vi "Act System RT main.vi"() -> ()   [LabVIEW 2014]
uses:
  <vilib>/myRIO/Instrument Drivers/Onboard IO/PWM/typedefs/PWM Reference.ctl
  <vilib>/myRIO/Common/Instrument Driver Framework/Utilities/typedefs/myRIO Generic Hardware Reference.ctl
  <vilib>/myRIO/Common/Instrument Driver Framework/Utilities/typedefs/Hardware Version Enum.ctl
  <vilib>/myRIO/Common/Instrument Driver Framework/Utilities/typedefs/myRIO v1.0 Reference.ctl
  <vilib>/myRIO/Common/Instrument Driver Framework/Utilities/typedefs/Generic FPGA Reference.ctl
  <vilib>/myRIO/Common/Instrument Driver Framework/myRIO v1.0/PWM/typedefs/PWM Channels Enum.ctl
  <vilib>/myRIO/Instrument Drivers/Onboard IO/PWM/typedefs/PWM Configuration.ctl
  <vilib>/userdefined/High Color/nirio_resource_hc.ctl
  <vilib>/myRIO/Instrument Drivers/Onboard IO/AI/typedefs/AI Reference.ctl
  <vilib>/myRIO/Common/Instrument Driver Framework/myRIO v1.0/AI/typedefs/AI Channels List.ctl
  <vilib>/myRIO/Common/Instrument Driver Framework/myRIO v1.0/AI/typedefs/AI Channels Enum.ctl
  <vilib>/myRIO/Common/Instrument Driver Framework/Utilities/typedefs/Analog Scaling Constants List.ctl
  <vilib>/myRIO/Common/Instrument Driver Framework/Utilities/typedefs/Analog Scaling Constants.ctl
  <vilib>/myRIO/Common/Instrument Driver Framework/myRIO v1.0/PWM/vis/myRIO v1.1 Open PWM.vi
  <vilib>/myRIO/Common/Instrument Driver Framework/myRIO v1.0/AI/vis/myRIO v1.1 Open AI.vi
  <vilib>/myRIO/Common/Instrument Driver Framework/Utilities/vis/Validate Channels.vi
  <vilib>/myRIO/Common/Instrument Driver Framework/myRIO v1.0/PWM/vis/myRIO v1.0 Reserve PWM.vi
  <vilib>/myRIO/Instrument Drivers/Onboard IO/PWM/vis/Set Duty Cycle and Frequency.vi
  <vilib>/myRIO/Common/Instrument Driver Framework/myRIO v1.0/AI/vis/myRIO v1.0 Reserve AI.vi
  <vilib>/myRIO/Common/Instrument Driver Framework/myRIO v1.0/DIO/vis/myRIO v1.1 Open DIO.vi
  <vilib>/myRIO/Common/Instrument Driver Framework/myRIO v1.0/PWM/vis/myRIO v1.0 Close PWM.vi
  <vilib>/myRIO/Common/Instrument Driver Framework/myRIO v1.0/AI/vis/myRIO v1.0 Close AI.vi
  <vilib>/myRIO/Common/Instrument Driver Framework/myRIO v1.0/DIO/vis/myRIO v1.0 Close DIO.vi
  <vilib>/myRIO/Common/Instrument Driver Framework/myRIO v1.0/PWM/vis/myRIO v1.0 Build MUX Configuration PWM.vi
  <vilib>/myRIO/Common/Instrument Driver Framework/myRIO v1.0/Resource Manager/vis/myRIO v1.0 Reserve Channel List.vi
  <vilib>/myRIO/Common/Instrument Driver Framework/myRIO v1.0/AI/vis/myRIO v1.0 Build MUX Configuration AI.vi
  <vilib>/myRIO/Common/Instrument Driver Framework/myRIO v1.0/DIO/vis/myRIO v1.0 Reserve DIO.vi
  <vilib>/myRIO/Common/Instrument Driver Framework/myRIO v1.0/PWM/vis/myRIO v1.0 Unreserve PWM.vi
  <vilib>/myRIO/Common/Instrument Driver Framework/myRIO v1.0/AI/vis/myRIO v1.0 Unreserve AI.vi
  <vilib>/myRIO/Common/Instrument Driver Framework/myRIO v1.0/DIO/vis/myRIO v1.0 Unreserve DIO.vi
  <vilib>/myRIO/Common/Instrument Driver Framework/myRIO v1.0/Resource Manager/vis/myRIO v1.0 Create Configuration List.vi
  <vilib>/myRIO/Common/Instrument Driver Framework/myRIO v1.0/Resource Manager/vis/myRIO v1.0 Reserve Channel.vi
  <vilib>/myRIO/Common/Instrument Driver Framework/myRIO v1.0/Resource Manager/vis/myRIO v1.0 Unreserve Channel.vi
  <vilib>/myRIO/Common/Instrument Driver Framework/myRIO v1.0/DIO/vis/myRIO v1.0 Build MUX Configuration DIO.vi
  <vilib>/myRIO/Common/Instrument Driver Framework/myRIO v1.0/Resource Manager/vis/myRIO v1.0 Unreserve Channel List.vi
  <vilib>/myRIO/Common/Instrument Driver Framework/myRIO v1.0/Resource Manager/vis/myRIO v1.0 Build Mutex Name.vi
  <vilib>/Utility/VariantDataType/GetNumericInfo.vi
  <vilib>/Utility/error.llb/Error Cluster From Error Code.vi
  <vilib>/myRIO/Common/Instrument Driver Framework/myRIO v1.0/myRIO v1.1 Open.vi
  <vilib>/myRIO/Common/Instrument Driver Framework/Utilities/vis/IO Manager.vi
  <vilib>/myRIO/Common/Instrument Driver Framework/Utilities/vis/Configuration Manager.vi
  <vilib>/myRIO/Common/Instrument Driver Framework/myRIO v1.0/Resource Manager/vis/myRIO v1.0 Configure IO.vi
  <vilib>/myRIO/Common/Instrument Driver Framework/myRIO v1.0/myRIO v1.0 Close.vi
  <vilib>/myRIO/Common/Instrument Driver Framework/myRIO v1.0/AI/vis/myRIO v1.0 Get Scaling Constants AI.vi
  <vilib>/myRIO/Common/Instrument Driver Framework/myRIO v1.0/PWM/vis/myRIO v1.0 Write PWM.vi
  <vilib>/myRIO/Common/Instrument Driver Framework/myRIO v1.0/PWM/vis/myRIO v1.0 Shutdown PWM.vi
  <vilib>/myRIO/Common/Instrument Driver Framework/myRIO v1.0/AI/vis/myRIO v1.0 Read AI.vi
  <vilib>/myRIO/Common/Instrument Driver Framework/myRIO v1.0/DIO/vis/myRIO v1.0 Write DIO.vi
  <vilib>/myRIO/Common/Instrument Driver Framework/myRIO v1.0/DIO/vis/myRIO v1.0 Shutdown DIO.vi
  <vilib>/myRIO/Instrument Drivers/Onboard IO/AI/vis/myRIO AI Open.xnode
  <vilib>/myRIO/Instrument Drivers/Onboard IO/PWM/vis/myRIO PWM Open.xnode
  <vilib>/myRIO/Instrument Drivers/Onboard IO/DIO/DIO.lvlib
  <vilib>/myRIO/Instrument Drivers/Onboard IO/AI/AI.lvlib
  <vilib>/myRIO/Instrument Drivers/Onboard IO/PWM/PWM.lvlib
  <vilib>/gmath/NI_Gmath.lvlib
panel:
  out "Pot Control On":bool
  in  "Keyboard/Pot":bool
  out "PropmotorInput":dbl
  out "ServoInput":dbl
  in  "Pot. Degrees":dbl[](array[numeric])
  out "Volts":dbl(knob) scale=0.0..10.0
  in  "Propmotor PWM Channel":tag="C/PWM1"
  in  "Servo PWM Channel":tag="C/PWM0"
  out "Propmotor keybd":dbl
  out "ServoKeybd":dbl
  out "error out":errorcluster={"status"=FALSE, "code"=-363018, "source"=""}
  out "RT FP LED":bool
  in  "Stop":bool
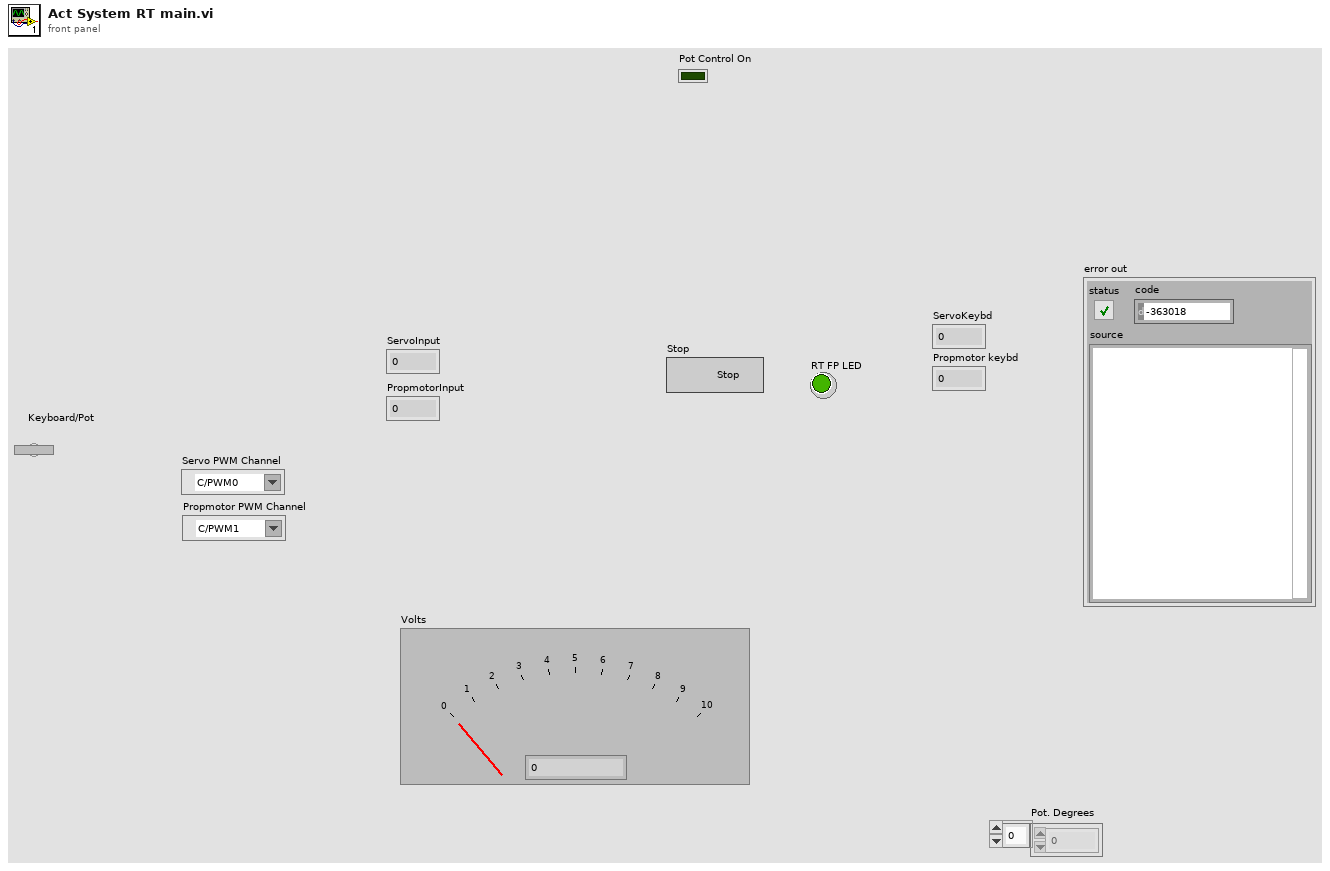
[diagram p1: front panel]
types:
  T1 = typedef "nirio_resource_hc.ctl" = tag
  T2 = typedef "Hardware Version Enum.ctl" = enum16{"Unknown", "myRIO-1900", "myRIO-1950"}
  T3 = typedef "PWM.lvlib/PWM Reference.ctl" = cluster{"myRIO Reference":T4, "PWM Channels Enum":T7, "PWM Configuration":T8}
  T4 = typedef "myRIO Generic Hardware Reference.ctl" = cluster{"myRIO Model":T2, "myRIO Hardware Reference":T5}
  T5 = typedef "myRIO v1.0 Reference.ctl" = cluster{"Generic FPGA Reference":T6, "Allow multiple opens":bool}
  T6 = typedef "Generic FPGA Reference.ctl" = refnum<k20>
  T7 = typedef "PWM Channels Enum.ctl" = enum16{"Not Connected", "C/PWM0", "C/PWM1", "A/PWM0", "A/PWM1", "A/PWM2", "B/PWM0", "B/PWM1", "B/PWM2"}
  T8 = typedef "PWM.lvlib/PWM Configuration.ctl" = cluster{"Frequency":dbl, "Duty Cycle":dbl}
  T9 = typedef "AI.lvlib/AI Reference.ctl" = cluster{"myRIO Reference":T4, "AI Channels List":T10, "AI Scaling Constants List":T12}
  T10 = typedef "AI Channels List.ctl" = T11[]
  T11 = typedef "AI Channels Enum.ctl" = enum16{"Not Connected", "AudioIn/Left", "AudioIn/Right", "C/AI0", "C/AI1", "A/AI0", "A/AI1", "A/AI2", "A/AI3", "B/AI0", "B/AI1", "B/AI2", "B/AI3"}
  T12 = typedef "Analog Scaling Constants List.ctl" = T13[]
  T13 = typedef "Analog Scaling Constants.ctl" = cluster{"LSB Weight (Volts)":dbl, "Offset (Volts)":dbl, "Signed?":bool}
  T14 = typedef "DIO.lvlib/DIO Reference.ctl" = cluster{"myRIO Reference":T4, "DIO Channels List":T15}
  T15 = typedef "DIO Channels List.ctl" = T16[]
  T16 = typedef "DIO Channels Enum.ctl" = enum16{"Not Connected", "C/DIO0", "C/DIO1", "C/DIO2", "C/DIO3", "C/DIO4", "C/DIO5", "C/DIO6", "C/DIO7", "A/DIO0", "A/DIO1", "A/DIO2", "A/DIO3", "A/DIO4", "A/DIO5", "A/DIO6", "A/DIO7", "A/DIO8", "A/DIO9", "A/DIO10", "A/DIO11", "A/DIO12", "A/DIO13", "A/DIO14", "A/DIO15", "B/DIO0", "B/DIO1", "B/DIO2", "B/DIO3", "B/DIO4", "B/DIO5", "B/DIO6", "B/DIO7", "B/DIO8", "B/DIO9", "B/DIO10", "B/DIO11", "B/DIO12", "B/DIO13", "B/DIO14", "B/DIO15", "LED0", "LED1", "LED2", "LED3", "Button0"}
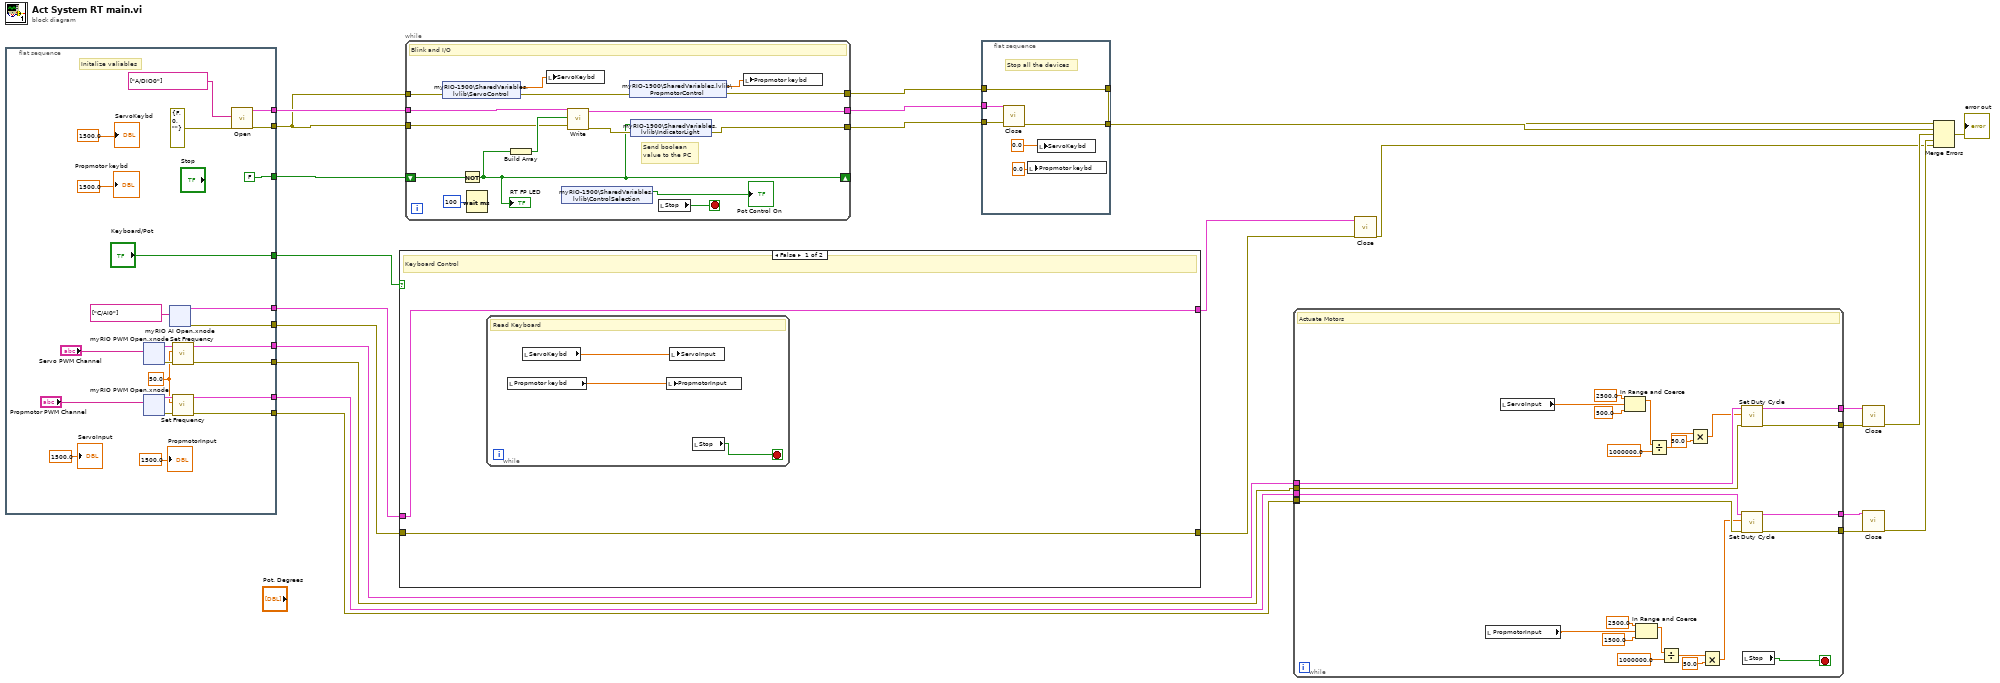
[diagram p0: block diagram]
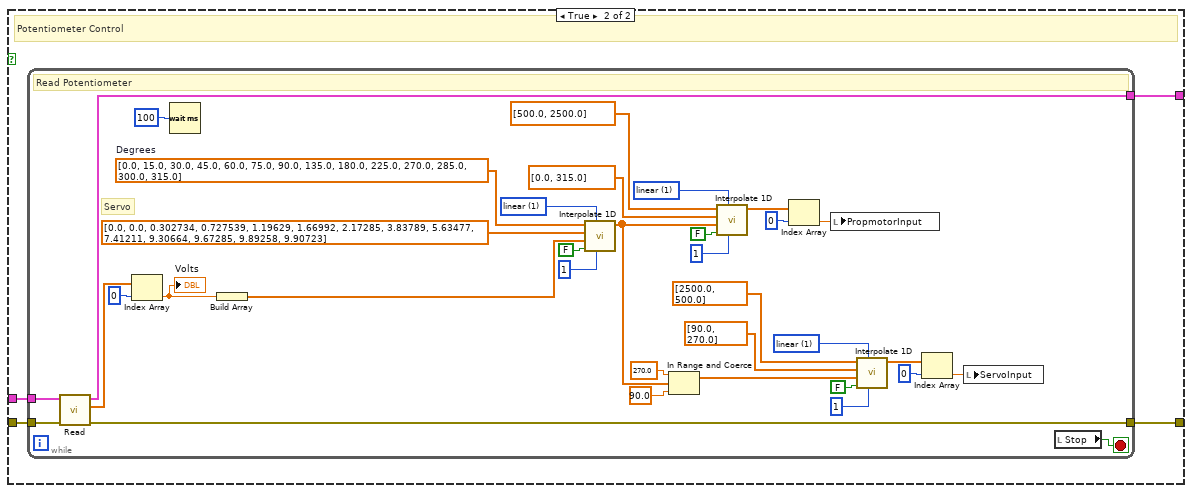
[diagram p2: hidden frame]
diagram:
  n1 = flat-sequence {
    tunnel: [FALSE] -> w25
    tunnel: [w48] -> w21
    tunnel: [w47] -> w24
    tunnel: [w34] -> w16
    tunnel: [w33] -> w15
    tunnel: [w32] -> w13
    tunnel: [w31] -> w12
    tunnel: [w30] -> w11
    tunnel: [w29] -> w14
    tunnel: ["Keyboard/Pot"] -> w1
    frame #0 {
      w35 = 50.0 ("Frequency [Hz]")
      # "Initalize valiables"
      n2 = xnode "myRIO PWM Open.xnode"("Channel Name"="Servo PWM Channel") -> ("error out"=w40:errorcluster, "PWM Ref Out"=w41:T3)  [unwired: 2 in]
      n3 = xnode "myRIO PWM Open.xnode"("Channel Name"="Propmotor PWM Channel") -> ("error out"=w37:errorcluster, "PWM Ref Out"=w38:T3)  [unwired: 2 in]
      n4 = xnode "myRIO AI Open.xnode"("Channel Names"=tag[] ["C/AI0"]) -> ("error out"=w33:errorcluster, "AI Ref Out"=w34:T9)  [unwired: 2 in]
      n5 = call <vilib>:"Set Frequency.vi"("error in (no error)"=w40, "Frequency [Hz]"=w35, "PWM Ref In"=w41) -> ("error out"=w32:errorcluster, "PWM Ref Out"=w29:T3)  [unwired: 6 in]
      n6 = call <vilib>:"Set Frequency.vi"("error in (no error)"=w37, "Frequency [Hz]"=w35, "PWM Ref In"=w38) -> ("error out"=w30:errorcluster, "PWM Ref Out"=w31:T3)  [unwired: 6 in]
      n7 = call <vilib>:"Open.vi"("error in (no error)"=errorcluster {"status"=FALSE, "code"=0, "source"=""}, "Channel Names"=tag[] ["A/DIO0"]) -> ("error out"=w48:errorcluster, "DIO Ref Out"=w47:T14)  [unwired: 8 in]
      "ServoKeybd" <- 1500.0
      "Propmotor keybd" <- 1500.0
      "ServoInput" <- 1500.0 ("ServoInput")
      "PropmotorInput" <- 1500.0 ("PropmotorInput")
    }
  }
  n8 = case shown="False" w1 {
    tunnel: w16 -> [w101 w108]
    tunnel: w15 -> [w100 w107]
    tunnel: [w101 w106] -> w4
    tunnel: [w100 w105] -> w3
    frame False {
      # "Keyboard Control"
      n9 = while {
        stop <- w102 stop-if-true
        # "Read Keyboard"
        n10 = local read "Propmotor keybd"() -> (w103:dbl)
        n11 = local read "ServoKeybd"() -> (w104:dbl)
        n12 = local write "PropmotorInput"(w103) -> ()
        n13 = local write "ServoInput"(w104) -> ()
        n14 = local read "Stop"() -> (w102:bool)
      }
    }
    frame True {
      # "Potentiometer Control"
      n15 = while {
        tunnel: w108 -> [w141]
        tunnel: w107 -> [w140]
        tunnel: [w137] -> w105
        tunnel: [w136] -> w106
        stop <- w142 stop-if-true
        w114 = 1 items=["nearest", "linear", "spline", "cubic Hermite", "Lagrange"] ("method")
        w126 = 1 items=["nearest", "linear", "spline", "cubic Hermite", "Lagrange"] ("method")
        w129 = dbl[] [0.0, 15.0, 30.0, 45.0, 60.0, 75.0, 90.0, 135.0, 180.0, 225.0, 270.0, 285.0, 300.0, 315.0]  # Degrees
        w131 = 1 items=["nearest", "linear", "spline", "cubic Hermite", "Lagrange"] ("method")
        # "Servo"
        # "Read Potentiometer"
        n16 = call <vilib>:"Read.vi"("error in (no error)"=w140, "AI Ref In"=w141) -> ("error out"=w137:errorcluster, "Values"=w139:dbl[], "AI Ref Out"=w136:T9)  [unwired: 7 in]
        n17 = Index Array(array=w139, index=0) -> (element=w134:dbl)
        "Volts" <- w134
        n18 = Wait (ms)(milliseconds to wait=u32 100) -> ()  [unwired: 1 out]
        n19 = Build Array(w134) -> (w133:dbl[])
        n20 = call <vilib>:"Interpolate 1D.vi"("ntimes"=1, "method"=w131, "X is monotonic"=FALSE, "xi"=w133, "X"=dbl[] [0.0, 0.0, 0.302734, 0.727539, 1.19629, 1.66992, 2.17285, 3.83789, 5.63477, 7.41211, 9.30664, 9.67285, 9.89258, 9.90723] ("VoltageIn"), "Y"=w129) -> ("yi"=w112:dbl[])  [unwired: 3 in, 2 out]
        n21 = In Range and Coerce(upper limit=270.0, x=w112, lower limit=90.0) -> (coerced(x)=w122:dbl[])  [unwired: 1 out]
        n22 = call <vilib>:"Interpolate 1D.vi"("ntimes"=1, "method"=w114, "X is monotonic"=FALSE, "xi"=w112, "X"=dbl[] [0.0, 315.0] ("X servo (degrees)"), "Y"=dbl[] [500.0, 2500.0] ("Y servo (PWM)")) -> ("yi"=w113:dbl[])  [unwired: 3 in, 2 out]
        n23 = Index Array(array=w113, index=0) -> (element=w109:dbl)
        n24 = local write "PropmotorInput"(w109) -> ()
        n25 = call <vilib>:"Interpolate 1D.vi"("ntimes"=1, "method"=w126, "X is monotonic"=FALSE, "xi"=w122, "X"=dbl[] [90.0, 270.0] ("X servo (degrees)"), "Y"=dbl[] [2500.0, 500.0] ("Y servo (PWM)")) -> ("yi"=w121:dbl[])  [unwired: 3 in, 2 out]
        n26 = Index Array(array=w121, index=0) -> (element=w110:dbl)
        n27 = local write "ServoInput"(w110) -> ()
        n28 = local read "Stop"() -> (w142:bool)
      }
    }
  }
  n29 = while {
    shift-right: [w151] -> _
    shift-left: w25 -> [w159]
    tunnel: w24 -> [w155]
    tunnel: w21 -> [w154]
    tunnel: [w152] -> w23
    tunnel: [w157] -> w22
    tunnel: [w149] -> w18
    tunnel: w21 -> [w148]
    stop <- w145 stop-if-true
    # "Send boolean\nvalue to the PC"
    # "Blink and I/O"
    n30 = shared-variable "myRIO-1900\\SharedVariables.lvlib\\ServoControl"(error in=w148) -> (w146:dbl, error out=w150:errorcluster)
    n31 = Not(x=w159) -> (.not. x?=w151:bool)
    "RT FP LED" <- w151
    n32 = Wait (ms)(milliseconds to wait=u32 100) -> ()  [unwired: 1 out]
    n33 = Build Array(w151) -> (w156:bool[])
    n34 = local write "ServoKeybd"(w146) -> ()
    n35 = shared-variable "myRIO-1900\\SharedVariables.lvlib\\ControlSelection"() -> (→"Pot Control On":bool)  [unwired: 1 in, 1 out]
    n36 = call <vilib>:"Write.vi"("error in (no error)"=w154, "Values"=w156, "DIO Ref In"=w155) -> ("error out"=w153:errorcluster, "DIO Ref Out"=w157:T14)  [unwired: 6 in]
    n37 = shared-variable "myRIO-1900\\SharedVariables.lvlib\\PropmotorControl"(error in=w150) -> (w147:dbl, error out=w149:errorcluster)
    n38 = shared-variable "myRIO-1900\\SharedVariables.lvlib\\IndicatorLight"(w151, error in=w153) -> (error out=w152:errorcluster)
    n39 = local read "Stop"() -> (w145:bool)
    n40 = local write "Propmotor keybd"(w147) -> ()
  }
  n41 = flat-sequence {
    tunnel: w23 -> [w165]
    tunnel: w22 -> [w164]
    tunnel: [w163] -> w20
    tunnel: w18 -> [w162]
    tunnel: [w162] -> w17
    frame #0 {
      # "Stop all the devices"
      n42 = call <vilib>:"Close.vi"("error in (no error)"=w165, "DIO Ref In"=w164) -> ("error out"=w163:errorcluster)  [unwired: 9 in]
      n43 = local write "Propmotor keybd"(0.0) -> ()
      n44 = local write "ServoKeybd"(0.0) -> ()
    }
  }
  n45 = while {
    tunnel: w14 -> [w189]
    tunnel: w13 -> [w188]
    tunnel: w12 -> [w187]
    tunnel: w11 -> [w186]
    tunnel: [w186] -> _
    tunnel: [w185] -> w8
    tunnel: [w184] -> w7
    tunnel: [w183] -> w5
    tunnel: [w182] -> w6
    stop <- w190 stop-if-true
    # "Actuate Motors"
    n46 = local read "PropmotorInput"() -> (w167:dbl)
    n47 = local read "ServoInput"() -> (w166:dbl)
    n48 = In Range and Coerce(upper limit=2500.0, x=w166, lower limit=500.0) -> (coerced(x)=w180:dbl)  [unwired: 1 out]
    n49 = In Range and Coerce(upper limit=2500.0, x=w167, lower limit=1500.0) -> (coerced(x)=w173:dbl)  [unwired: 1 out]
    n50 = Divide(x=w180, y=1000000.0) -> (x/y=w178:dbl)
    n51 = Divide(x=w173, y=1000000.0) -> (x/y=w170:dbl)
    n52 = Multiply(x=w178, y=50.0) -> (x*y=w168:dbl)
    n53 = Multiply(x=w170, y=50.0) -> (x*y=w169:dbl)
    n54 = call <vilib>:"Set Duty Cycle.vi"("error in (no error)"=w188, "Duty Cycle"=w168, "PWM Ref In"=w189) -> ("error out"=w184:errorcluster, "PWM Ref Out"=w185:T3)  [unwired: 6 in]
    n55 = call <vilib>:"Set Duty Cycle.vi"("error in (no error)"=w186, "Duty Cycle"=w169, "PWM Ref In"=w187) -> ("error out"=w183:errorcluster, "PWM Ref Out"=w182:T3)  [unwired: 6 in]
    n56 = local read "Stop"() -> (w190:bool)
  }
  n57 = call <vilib>:"Close.vi"("error in (no error)"=w3, "AI Ref In"=w4) -> ("error out"=w2:errorcluster)  [unwired: 9 in]
  n58 = call <vilib>:"Close.vi"("error in (no error)"=w7, "PWM Ref In"=w8) -> ("error out"=w9:errorcluster)  [unwired: 9 in]
  n59 = call <vilib>:"Close.vi"("error in (no error)"=w5, "PWM Ref In"=w6) -> ("error out"=w10:errorcluster)  [unwired: 9 in]
  n60 = Merge Errors(w17, w20, w9, w10, w2) -> (→"error out":errorcluster)
